vi "SpecAn Configure ACP.vi"(0 "Instrument Handle In":refnum<k21>, 1 "Selector String":string, 5 "ACP Configuration":T1={"Power Units"=0, "Averaging Enabled"=0, "Averaging Count"=10, "Averaging Type"=0, "FFT Window"=1, "FFT Padding"=1.0, "RBW Auto"=1, "RBW (Hz)"=10000.0, "RBW Filter Type"=1, "Sweep Time Auto"=1, "Sweep Time Interval (s)"=0.001, "Component Carrier Configuration"=[{"Frequency (Hz)"=0.0, "Integration Bandwidth (Hz)"=18000000.0, "Mode"=1, "RRC Filter Enabled"=1, "RRC Alpha"=0.22}], "Offset Channel Configuration"=[{"Integration Bandwidth (Hz)"=18000000.0, "Enabled"=1, "Frequency (Hz)"=20000000.0, "Sideband"=2, "Power Reference Carrier"=0, "Power Reference Specific Index"=0, "Relative Attenuation (dB)"=0.0, "RRC Filter Enabled"=0, "RRC Alpha"=0.22}]} {"Offset Channel Configuration"."RRC Alpha" format="%.3g"; "Offset Channel Configuration"."RRC Filter Enabled" items=["False", "True"]; "Offset Channel Configuration"."Relative Attenuation (dB)" format="%.2f"; "Offset Channel Configuration"."Power Reference Carrier" items=["Closest", "Highest", "Composite", "Specific"]; "Offset Channel Configuration"."Sideband" items=["Neg", "Pos", "Both"]; "Offset Channel Configuration"."Frequency (Hz)" format="%.3p"; "Offset Channel Configuration"."Enabled" items=["False", "True"]; "Offset Channel Configuration"."Integration Bandwidth (Hz)" format="%.3p"; "Component Carrier Configuration"."RRC Alpha" format="%.3g"; "Component Carrier Configuration"."RRC Filter Enabled" items=["False", "True"]; "Component Carrier Configuration"."Mode" items=["Passive", "Active"]; "Component Carrier Configuration"."Frequency (Hz)" format="%.3p"; "Component Carrier Configuration"."Integration Bandwidth (Hz)" format="%.3p"; "Sweep Time Interval (s)" format="%.2p"; "Sweep Time Auto" items=["False", "True"]; "RBW Filter Type" items=["FFT Based", "Gaussian", "Flat", "Synch Tuned - 4", "Synch Tuned - 5"]; "RBW (Hz)" format="%.3p"; "RBW Auto" items=["False", "True"]; "FFT Padding" format="%.2f"; "FFT Window" items=["None", "Flat Top", "Hanning", "Hamming", "Gaussian", "Blackman", "Blackman-Harris", "Kaiser-Bessel"]; "Averaging Type" items=["RMS", "Log", "Scalar", "Max", "Min", "Vector"]; "Averaging Enabled" items=["False", "True"]; "Power Units" items=["dBm", "dBm/Hz"]}, 11 "error in (no error)":errorcluster) -> (4 "Instrument Handle Out":refnum<k21>, 15 "error out":errorcluster)   [LabVIEW 2019, in "RFmxSpecAn.lvlib"]
doc: "Configures common settings for the ACP measurement and selects the measurement."
uses:
  RFmxSpecAn.lvlib
  Typedefs/SpecAn ACP Configuration.ctl
  Typedefs/SpecAn ACP Component Carrier Configuration.ctl
  Typedefs/SpecAn ACP Offset Channel Configuration.ctl
  <vilib>/RFmx/SpecAn/mx/RFmxSpecAn.llb/RFmxSpecAn Build Signal String.vi
  <vilib>/RFmx/RFInstr/mx/RFmxInstr.llb/RFmxInstr Build Signal String.vi
  <vilib>/RFmx/SpecAn/mx/RFmxSpecAn.llb/RFmxSpecAn Select Measurement (Single).vi
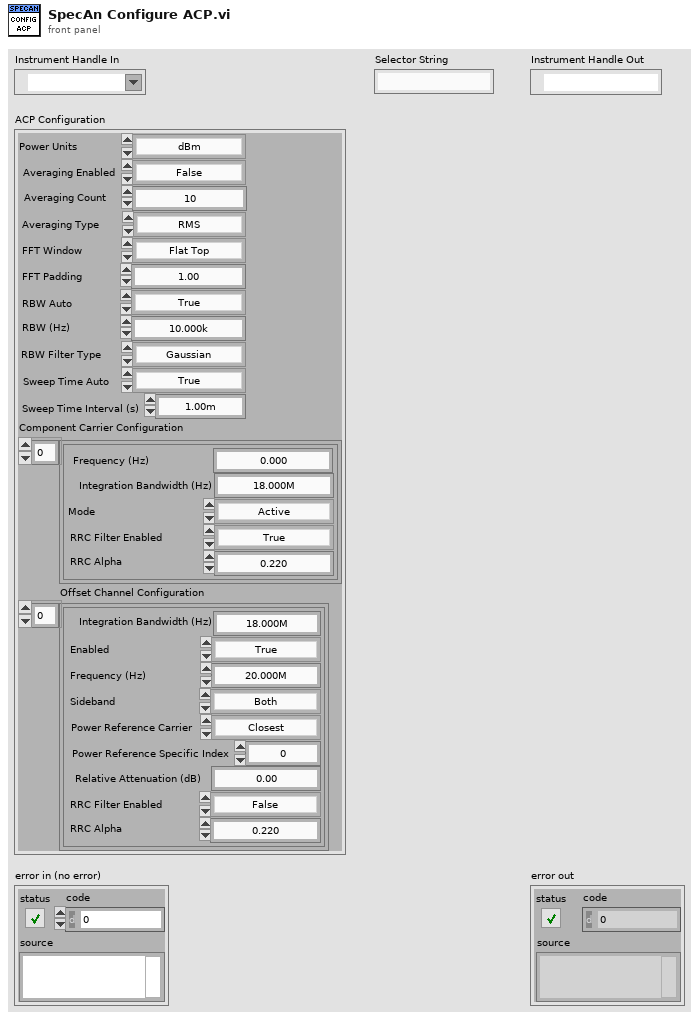
[diagram p1: front panel]
types:
  T1 = typedef "RFmxSpecAn.lvlib/SpecAn ACP Configuration.ctl" = cluster{"Power Units":i32, "Averaging Enabled":i32, "Averaging Count":i32, "Averaging Type":i32, "FFT Window":i32, "FFT Padding":dbl, "RBW Auto":i32, "RBW (Hz)":dbl, "RBW Filter Type":i32, "Sweep Time Auto":i32, "Sweep Time Interval (s)":dbl, "Component Carrier Configuration":T2[], "Offset Channel Configuration":T3[]}
  T2 = typedef "RFmxSpecAn.lvlib/SpecAn ACP Component Carrier Configuration.ctl" = cluster{"Frequency (Hz)":dbl, "Integration Bandwidth (Hz)":dbl, "Mode":i32, "RRC Filter Enabled":i32, "RRC Alpha":dbl}
  T3 = typedef "RFmxSpecAn.lvlib/SpecAn ACP Offset Channel Configuration.ctl" = cluster{"Integration Bandwidth (Hz)":dbl, "Enabled":i32, "Frequency (Hz)":dbl, "Sideband":i32, "Power Reference Carrier":i32, "Power Reference Specific Index":i32, "Relative Attenuation (dB)":dbl, "RRC Filter Enabled":i32, "RRC Alpha":dbl}
  T4 = enum16{"ACP", "CCDF", "CHP", "FCnt", "Harmonics", "OBW", "SEM", "Spectrum", "Spur", "TXP", "AMPM", "DPD", "IQ", "IM", "NF", "PhaseNoise", "PAVT"}
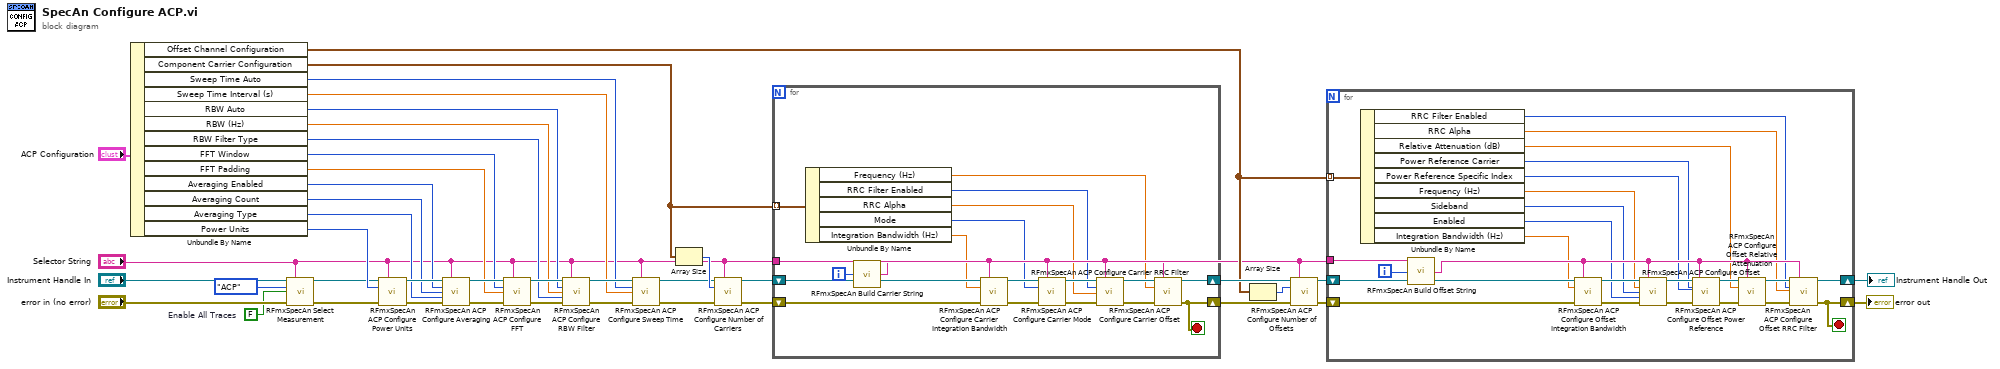
[diagram p0: block diagram]
diagram:
  w1 = FALSE  # Enable All Traces
  n1 = Unbundle By Name("ACP Configuration") -> ("Offset Channel Configuration"=w5:T3[], "Component Carrier Configuration"=w9:T2[], "Sweep Time Auto"=w16:i32, "Sweep Time Interval (s)"=w15:dbl, "RBW Auto"=w17:i32, "RBW (Hz)"=w18:dbl, "RBW Filter Type"=w19:i32, "FFT Window"=w21:i32, "FFT Padding"=w20:dbl, "Averaging Enabled"=w24:i32, "Averaging Count"=w23:i32, "Averaging Type"=w22:i32, "Power Units"=w25:i32)
  n2 = call-poly <vilib>:"RFmxSpecAn Select Measurement.vi"("Instrument Handle In"="Instrument Handle In", "Selector String"="Selector String", "Measurement"=T4."ACP", "Enable All Traces"=w1, "error in (no error)"="error in (no error)") -> ("Instrument Handle Out"=w13:refnum<k21>, "error out"=w37:errorcluster)  [unwired: 9 in]
  n3 = call <vilib>:"RFmxSpecAn ACP Configure Power Units.vi"("Instrument Handle In"=w13, "Selector String"="Selector String", "Power Units"=w25, "error in (no error)"=w37) -> ("Instrument Handle Out"=w29:refnum<k21>, "error out"=w38:errorcluster)  [unwired: 10 in]
  n4 = call <vilib>:"RFmxSpecAn ACP Configure Averaging.vi"("Instrument Handle In"=w29, "Selector String"="Selector String", "Averaging Enabled"=w24, "Averaging Count"=w23, "Averaging Type"=w22, "error in (no error)"=w38) -> ("Instrument Handle Out"=w28:refnum<k21>, "error out"=w41:errorcluster)  [unwired: 8 in]
  n5 = call <vilib>:"RFmxSpecAn ACP Configure FFT.vi"("Instrument Handle In"=w28, "Selector String"="Selector String", "FFT Window"=w21, "FFT Padding"=w20, "error in (no error)"=w41) -> ("Instrument Handle Out"=w30:refnum<k21>, "error out"=w39:errorcluster)  [unwired: 9 in]
  n6 = call <vilib>:"RFmxSpecAn ACP Configure RBW Filter.vi"("Instrument Handle In"=w30, "Selector String"="Selector String", "RBW Auto"=w17, "RBW (Hz)"=w18, "RBW Filter Type"=w19, "error in (no error)"=w39) -> ("Instrument Handle Out"=w27:refnum<k21>, "error out"=w40:errorcluster)  [unwired: 8 in]
  n7 = call <vilib>:"RFmxSpecAn ACP Configure Sweep Time.vi"("Instrument Handle In"=w27, "Selector String"="Selector String", "Sweep Time Auto"=w16, "Sweep Time Interval (s)"=w15, "error in (no error)"=w40) -> ("Instrument Handle Out"=w11:refnum<k21>, "error out"=w36:errorcluster)  [unwired: 9 in]
  n8 = Array Size(array=w9) -> (size(s)=w12:i32)
  n9 = call <vilib>:"RFmxSpecAn ACP Configure Number of Carriers.vi"("Instrument Handle In"=w11, "Selector String"="Selector String", "Number of Carriers"=w12, "error in (no error)"=w36) -> ("Instrument Handle Out"=w10:refnum<k21>, "error out"=w35:errorcluster)  [unwired: 10 in]
  n10 = for {
    tunnel: w9 -> [w51] mode=indexing
    shift-right: [w56] -> w33
    shift-left: w35 -> [w60]
    shift-right: [w50] -> w6
    shift-left: w10 -> [w55]
    tunnel: "Selector String" -> [w43]
    i -> [w49]
    stop <- w56 stop-if-true
    n11 = Unbundle By Name(w51) -> ("Frequency (Hz)"=w48:dbl, "RRC Filter Enabled"=w47:i32, "RRC Alpha"=w46:dbl, "Mode"=w45:i32, "Integration Bandwidth (Hz)"=w44:dbl)
    n12 = call <vilib>:"RFmxSpecAn Build Carrier String.vi"("Signal Name"=w43, "Carrier Number"=w49) -> ("Carrier String"=w42:string)  [unwired: 13 in]
    n13 = call <vilib>:"RFmxSpecAn ACP Configure Carrier Integration Bandwidth.vi"("Instrument Handle In"=w55, "Selector String"=w42, "Integration Bandwidth (Hz)"=w44, "error in (no error)"=w60) -> ("Instrument Handle Out"=w54:refnum<k21>, "error out"=w59:errorcluster)  [unwired: 10 in]
    n14 = call <vilib>:"RFmxSpecAn ACP Configure Carrier Mode.vi"("Instrument Handle In"=w54, "Selector String"=w42, "Carrier Mode"=w45, "error in (no error)"=w59) -> ("Instrument Handle Out"=w53:refnum<k21>, "error out"=w58:errorcluster)  [unwired: 10 in]
    n15 = call <vilib>:"RFmxSpecAn ACP Configure Carrier RRC Filter.vi"("Instrument Handle In"=w53, "Selector String"=w42, "RRC Filter Enabled"=w47, "RRC Alpha"=w46, "error in (no error)"=w58) -> ("Instrument Handle Out"=w52:refnum<k21>, "error out"=w57:errorcluster)  [unwired: 9 in]
    n16 = call <vilib>:"RFmxSpecAn ACP Configure Carrier Offset.vi"("Instrument Handle In"=w52, "Selector String"=w42, "Carrier Frequency (Hz)"=w48, "error in (no error)"=w57) -> ("Instrument Handle Out"=w50:refnum<k21>, "error out"=w56:errorcluster)  [unwired: 10 in]
  }
  n17 = Array Size(array=w5) -> (size(s)=w7:i32)
  n18 = call <vilib>:"RFmxSpecAn ACP Configure Number of Offsets.vi"("Instrument Handle In"=w6, "Selector String"="Selector String", "Number of Offsets"=w7, "error in (no error)"=w33) -> ("Instrument Handle Out"=w8:refnum<k21>, "error out"=w34:errorcluster)  [unwired: 10 in]
  n19 = for {
    tunnel: w5 -> [w79] mode=indexing
    shift-right: [w80] -> w32
    shift-left: w34 -> [w85]
    shift-right: [w73] -> w4
    shift-left: w8 -> [w78]
    tunnel: "Selector String" -> [w61]
    i -> [w72]
    stop <- w80 stop-if-true
    n20 = Unbundle By Name(w79) -> ("RRC Filter Enabled"=w70:i32, "RRC Alpha"=w69:dbl, "Relative Attenuation (dB)"=w68:dbl, "Power Reference Carrier"=w67:i32, "Power Reference Specific Index"=w66:i32, "Frequency (Hz)"=w65:dbl, "Sideband"=w64:i32, "Enabled"=w63:i32, "Integration Bandwidth (Hz)"=w62:dbl)
    n21 = call <vilib>:"RFmxSpecAn Build Offset String.vi"("Signal Name"=w61, "Offset Number"=w72) -> ("Offset String"=w71:string)  [unwired: 13 in]
    n22 = call <vilib>:"RFmxSpecAn ACP Configure Offset Integration Bandwidth.vi"("Instrument Handle In"=w78, "Selector String"=w71, "Integration Bandwidth (Hz)"=w62, "error in (no error)"=w85) -> ("Instrument Handle Out"=w77:refnum<k21>, "error out"=w84:errorcluster)  [unwired: 10 in]
    n23 = call <vilib>:"RFmxSpecAn ACP Configure Offset.vi"("Instrument Handle In"=w77, "Selector String"=w71, "Offset Frequency (Hz)"=w65, "Offset Sideband"=w64, "Offset Enabled"=w63, "error in (no error)"=w84) -> ("Instrument Handle Out"=w76:refnum<k21>, "error out"=w83:errorcluster)  [unwired: 8 in]
    n24 = call <vilib>:"RFmxSpecAn ACP Configure Offset Power Reference.vi"("Instrument Handle In"=w76, "Selector String"=w71, "Offset Power Reference Carrier"=w67, "Offset Power Reference Specific"=w66, "error in (no error)"=w83) -> ("Instrument Handle Out"=w75:refnum<k21>, "error out"=w82:errorcluster)  [unwired: 9 in]
    n25 = call <vilib>:"RFmxSpecAn ACP Configure Offset Relative Attenuation.vi"("Instrument Handle In"=w75, "Selector String"=w71, "Relative Attenuation (dB)"=w68, "error in (no error)"=w82) -> ("Instrument Handle Out"=w74:refnum<k21>, "error out"=w81:errorcluster)  [unwired: 10 in]
    n26 = call <vilib>:"RFmxSpecAn ACP Configure Offset RRC Filter.vi"("Instrument Handle In"=w74, "Selector String"=w71, "RRC Filter Enabled"=w70, "RRC Alpha"=w69, "error in (no error)"=w81) -> ("Instrument Handle Out"=w73:refnum<k21>, "error out"=w80:errorcluster)  [unwired: 9 in]
  }
  "Instrument Handle Out" <- w4
  "error out" <- w32
